vi "ReverseRow2DArray.vi"(1 "2DArray_in":dbl[][](array[numeric])) -> (0 "2DArray_out":dbl[][](array[numeric]))   [LabVIEW 2013]
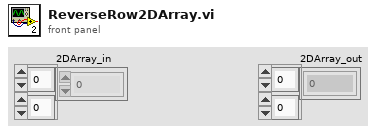
[diagram p1: front panel]
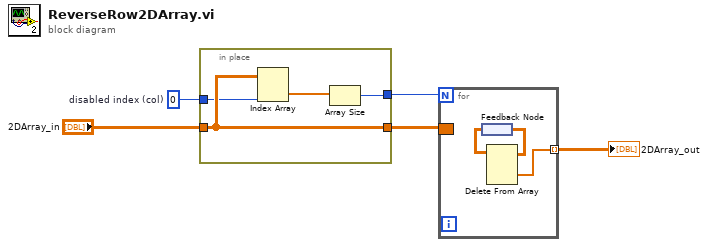
[diagram p0: block diagram]
diagram:
  w4 = 0  # disabled index (col)
  n1 = in-place {
    in-place-border: "2DArray_in" -> [w9]
    in-place-border: [w9] -> w2
    in-place-border: w4 -> [w8]
    in-place-border: [w6] -> w1
    n2 = Index Array(array=w9, index (col)=w8) -> (element=w7:dbl[])  [unwired: 1 in]
    n3 = Array Size(array=w7) -> (size(s)=w6:i32)
  }
  n4 = for {
    N: w1 -> [_]
    tunnel: [w12] -> w3 mode=indexing
    border: w2 -> [_]
    n5 = feedback #1() -> (w11:dbl[][])
    n6 = Delete From Array(array=w11) -> (deleted portion=w12:dbl[], array with subset deleted=w10:dbl[][])  [unwired: 3 in]
    n7 = feedback-in #1(w10) -> ()
  }
  "2DArray_out" <- w3
